vi "connect_TCP.vi"(4 "error in":errorcluster, 7 "deviceAddress":string) -> (0 "error ECC_connect":errorcluster, 3 "connection ID":refnum<k5>)   [LabVIEW 2016, in "AMC_VIs.lvlib"]
doc: "Initializes and connects the selected ECC (0..n).\nThis has to be done before any other function (except ECC_Check and ECC_ReleaseInfo) can be called.\nThe returned handle is used to address the device in further communication.\n\nInput\n deviceAddress IP address of the device\n error error message\n\nOutput\n connection ID ID that identifies the connection to a certain device\n error error message\n\n* required inputs"
uses:
  AMC_VIs.lvlib
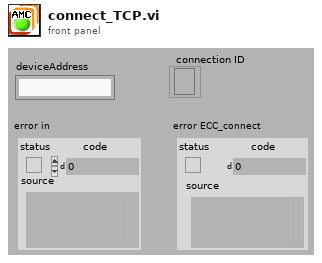
[diagram p1: front panel]
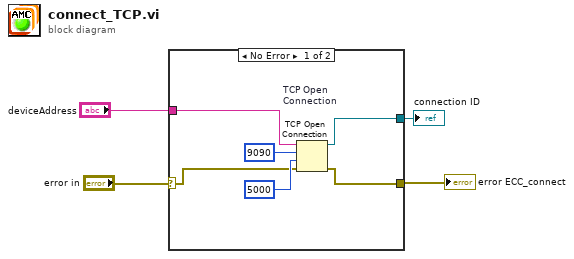
[diagram p0: block diagram]
diagram:
  n1 = case shown="No Error" "error in" {
    selector: "error in" -> [w6 w11]
    tunnel: "deviceAddress" -> [w5 _]
    tunnel: [w8 _] -> w1
    tunnel: [w7 w11] -> w2
    frame No Error {
      n2 = TCP Open Connection "TCP Open \nConnection"(address=w5, remote port or service name=u16 9090 ("port"), timeout ms (60000)=5000 ("timeout ms (25000)"), error in (no error)=w6) -> (connection ID=w8:refnum<k5>, error out=w7:errorcluster)  [unwired: 1 in]
    }
    frame Error {
    }
  }
  "error ECC_connect" <- w2
  "connection ID" <- w1
